vi "Build Graph.vi"(10 "Numeric":dbl, 11 "Reset Graph":bool) -> (2 "Array":dbl[](array[numeric]))   [LabVIEW 2017]
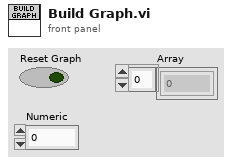
[diagram p1: front panel]
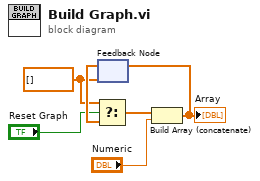
[diagram p0: block diagram]
diagram:
  w4 = dbl[] []
  n1 = feedback #1(w4) -> (w6:dbl[])
  n2 = Select(t=w4, s="Reset Graph", f=w6) -> (s? t:f=w2:dbl[])
  n3 = Build Array (concatenate)(w2, "Numeric") -> (w5:dbl[])
  "Array" <- w5
  n4 = feedback-in #1(w5) -> ()
